vi "3. FGV Machine number.vi"(0 "VISA resource name":refnum<visa-resource-name>="COM3", 11 "error in (no error)":errorcluster) -> (4 "Machine":i32, 10 "Checksum":u32, 15 "error out":errorcluster)   [LabVIEW 2014]
uses:
  control/FGV Serial Tasks.ctl
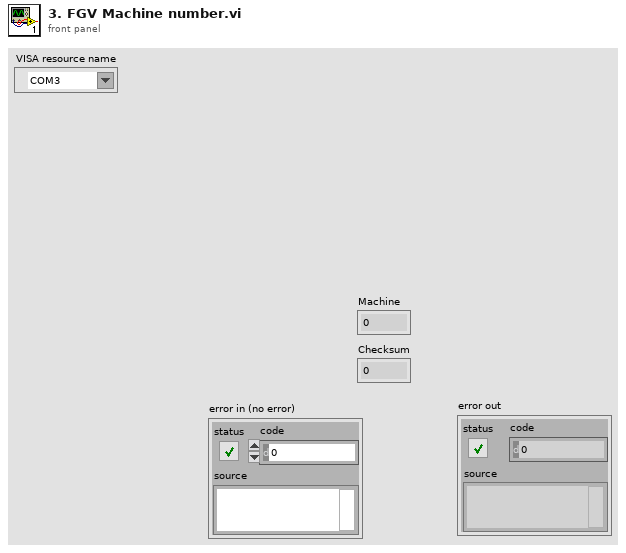
[diagram p1: front panel]
types:
  T1 = typedef "FGV Serial Tasks.ctl" = enum16{"Open", "Read", "Write", "Close", "Flush"}
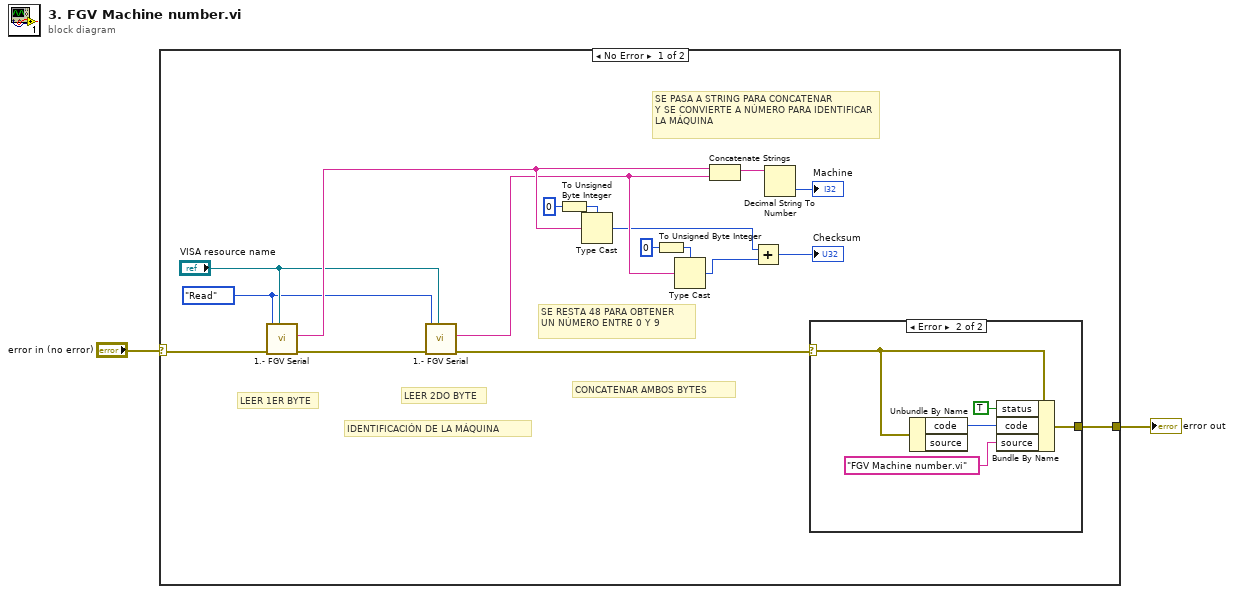
[diagram p0: block diagram]
diagram:
  n1 = case shown="No Error" "error in (no error)" {
    selector: "error in (no error)" -> [w14 w26]
    tunnel: [w17 w26] -> w1
    frame No Error {
      w3 = FGV_Serial_Tasks."Read" ("Task")
      # "SE PASA A STRING PARA CONCATENAR\nY SE CONVIERTE A NÚMERO PARA IDENTIFICAR LA MÁQUINA"
      # "SE RESTA 48 PARA OBTENER\nUN NÚMERO ENTRE 0 Y 9"
      # "CONCATENAR AMBOS BYTES"
      # "LEER 2DO BYTE"
      # "LEER 1ER BYTE"
      # "IDENTIFICACIÓN DE LA MÁQUINA"
      n2 = call "1.- FGV Serial.vi"("VISA resource name"="VISA resource name", "error in (no error)"=w14, "Task"=w3) -> ("error out"=w19:errorcluster, "Receive buffer"=w16:string)  [unwired: 6 in, 1 out]
      n3 = call "1.- FGV Serial.vi"("VISA resource name"="VISA resource name", "error in (no error)"=w19, "Task"=w3) -> ("error out"=w18:errorcluster, "Receive buffer"=w15:string)  [unwired: 6 in, 1 out]
      n4 = To Unsigned Byte Integer(number=u8 0) -> (unsigned 8bit integer=w6:u8)
      n5 = Type Cast(type=w6, x=w16) -> (*(type *) &x=w5:u8)
      n6 = To Unsigned Byte Integer(number=u8 0) -> (unsigned 8bit integer=w9:u8)
      n7 = Type Cast(type=w9, x=w15) -> (*(type *) &x=w4:u8)
      n8 = Concatenate Strings(w16, w15) -> (w12:string)
      n9 = Add(x=w5, y=w4) -> (x+y=→"Checksum":u8)
      n10 = Decimal String To Number(string=w12) -> (number=→"Machine":i32)  [unwired: 2 in, 1 out]
      n11 = case shown="Error" w18 {
        selector: w18 -> [w20 w24]
        tunnel: [w20 w23] -> w17
        frame No Error {
        }
        frame Error {
          n12 = Unbundle By Name(w24) -> ("code"=w25:i32)  [unwired: 1 out]
          n13 = Bundle By Name(cluster=w24, "status"=TRUE, "code"=w25, "source"="FGV Machine number.vi") -> (w23:errorcluster)
        }
      }
    }
    frame Error {
    }
  }
  "error out" <- w1
